vi "PCO_SetFlimPhaseSequenceParameter.vi"(0 "ph":u64, 1 "wTapSelect":u16(ring) items=["Tap A+B", "Tap A", "Tap B"], 5 "wPhaseNumber":u16(ring) items=["shiftablePair", "2", "4", "8", "16"], 7 "wPhaseSymmetry":u16(ring) items=["no", "yes"], 9 "wPhaseOrder":u16(ring) items=["ascending", "opposite"], 11 "error in (no error)":errorcluster {"code" format="%x"}) -> (4 "ph out":u64, 6 "ErrorMessage":i32 format="%x", 15 "error out":errorcluster {"code" format="%x"})   [LabVIEW 2019, in "SDK.lvlib" / "SpecialCommandsFlim.lvlib"]
doc: "<b>Description:</b>\nSet configuration for the generation of phase image sequences. The combination of the described options determines the resulting length and sorting of phase sequences. One phase sequence is a sequence of single (phase) images covering a modulation period of 360°. A PCO_ArmCamera is required to update these settings.\n\n<b>Supported camera type:</b>\npco.flim\n\n<b>Descriptor dependency:</b>\nNone"
uses:
  SpecialCommandsFlim.lvlib
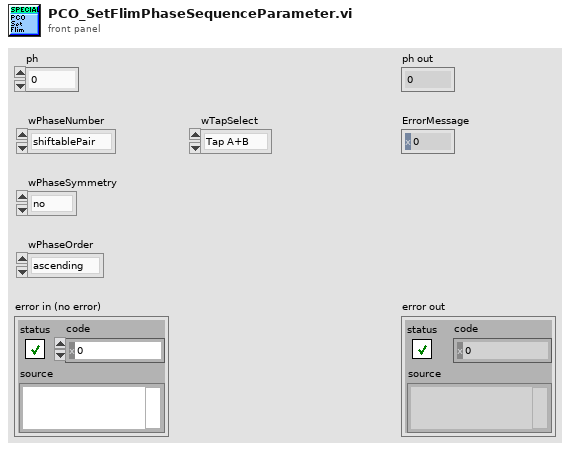
[diagram p1: front panel]
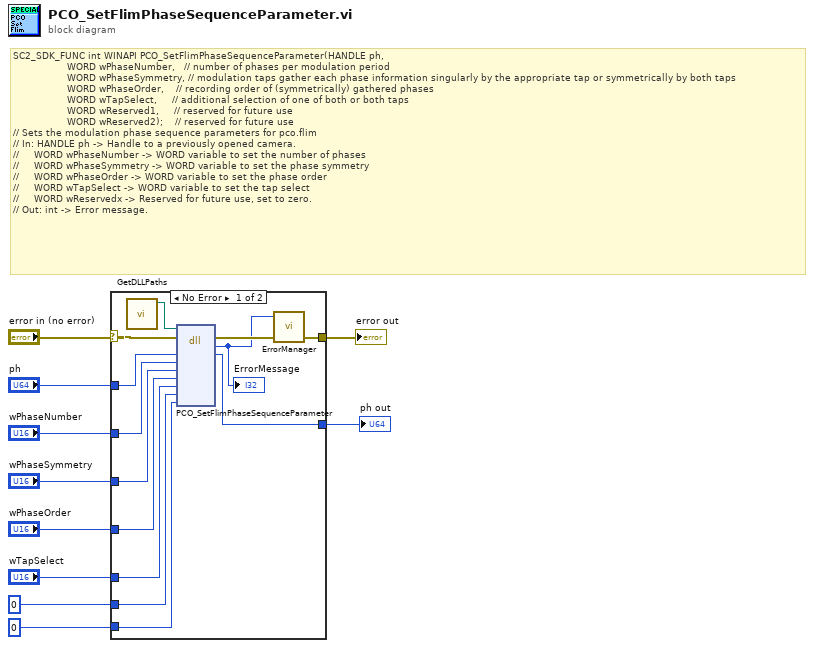
[diagram p0: block diagram]
diagram:
  # "SC2_SDK_FUNC int WINAPI PCO_SetFlimPhaseSequenceParameter(HANDLE ph, \n                  WORD wPhaseNumber,   // number of phases per modulation period\n                  WORD wPhaseSymmetry, // modulation taps gather each phase information singularly by the appropriate tap or symmetrically by both taps\n                  WORD wPhaseOrder,    // recording order of (symmetrically) gathered phases\n                  WORD wTapSelect,     // additional selection of one of both or both taps\n                  WORD wReserved1,     // reserved for future use\n                  WORD wReserved2);    // reserved for future use\n// Sets the modulation phase sequence parameters for pco.flim\n// In: HANDLE ph -> Handle to a previously opened camera.\n//     WORD wPhaseNumber -> WORD variable to set the number of phases\n//     WORD wPhaseSymmetry -> WORD variable to set the phase symmetry\n//     WORD wPhaseOrder -> WORD variable to set the phase order\n//     WORD wTapSelect -> WORD variable to set the tap select\n//     WORD wReservedx -> Reserved for future use, set to zero.\n// Out: int -> Error message."
  n1 = case shown="No Error" "error in (no error)" {
    selector: "error in (no error)" -> [w15 w25]
    tunnel: "ph" -> [w23 w24]
    tunnel: [w22 w24] -> w9
    tunnel: "wPhaseNumber" -> [w21 _]
    tunnel: "wPhaseSymmetry" -> [w20 _]
    tunnel: "wPhaseOrder" -> [w19 _]
    tunnel: "wTapSelect" -> [w18 _]
    tunnel: [w14 w25] -> w4
    tunnel: u16 0 ("wReserved1") -> [w17 _]
    tunnel: u16 0 ("wReserved1") -> [w16 _]
    frame No Error {
      n2 = call "GetDLLPaths.vi"() -> ("SC2_Cam_Path"=w11:path)  [unwired: 8 in, 3 out]
      n3 = dll-call lib="?" fn="PCO_SetFlimPhaseSequenceParameter"(path in=w11, error in=w15, "ph"=w23, "wPhaseNumber"=w21, "wPhaseSymmetry"=w20, "wPhaseOrder"=w19, "wTapSelect"=w18, "wReserved1"=w17, "wReserved2"=w16) -> (error out=w13:errorcluster, "return type"=w12:i32, "ph"=w22:u64)  [unwired: 7 in, 1 out]
      "ErrorMessage" <- w12
      n4 = call "ErrorManager.vi"("error in (no error)"=w13, "error code"=w12) -> ("error out"=w14:errorcluster)  [unwired: 2 in, 1 out]
    }
    frame Error {
    }
  }
  "ph out" <- w9
  "error out" <- w4
